vi "Write Objects.vi"(9 "Analyze Results Fluence.lvclass":refnum<class "Analyze Results Fluence.lvclass">, 10 "Analyze Results Energy Obj":refnum<class "Analyze Results Energy.lvclass">, 11 "Analyze Results Fluence and Energy in":refnum<class "Analyze Results Fluence and Energy.lvclass">) -> (3 "Analyze Results Fluence and Energy out":refnum<class "Analyze Results Fluence and Energy.lvclass">)   [LabVIEW 2014, in "Analyze Results Fluence and Energy.lvclass"]
uses:
  Analyze Results Fluence and Energy.lvclass
  JETI200 Overview and ShotID/HIJ Vision/Analyze/Results and Overlays/Results Energy/Analyze Results Energy.lvclass
  JETI200 Overview and ShotID/HIJ Vision/Analyze/Results and Overlays/Results Fluence/Analyze Results Fluence.lvclass
  Analyze Results Fluence and Energy.lvclass/Analyze Results Fluence and Energy.ctl
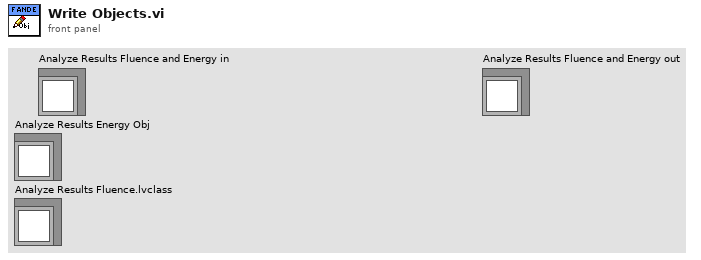
[diagram p1: front panel]
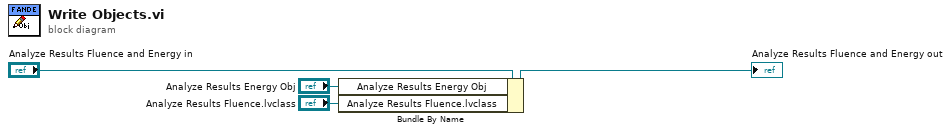
[diagram p0: block diagram]
diagram:
  n1 = Bundle By Name(cluster="Analyze Results Fluence and Energy in", "Analyze Results Energy Obj"="Analyze Results Energy Obj", "Analyze Results Fluence.lvclass"="Analyze Results Fluence.lvclass") -> (→"Analyze Results Fluence and Energy out":refnum<class "Analyze Results Fluence and Energy.lvclass">)
